vi "Move Stage.vi"(8 "error in (no error)":errorcluster, 9 "Y Axis":dbl, 10 "X Axis":dbl, 11 "2-Axis Stage in":refnum<class "XY Stage Process.lvclass">) -> (0 "error out":errorcluster, 3 "2-Axis Stage out":refnum<class "XY Stage Process.lvclass">)   [LabVIEW 2022 SP3, in "XY Stage Process.lvlib" / "XY Stage Process.lvclass"]
uses:
  XY Stage Process.lvclass
  XY Stage Process.lvclass/XY Stage Process.ctl
  Axis Objects/iMotion Controller/iMotion Controller.lvclass
  Process Framework/Process State Data/Process State Data.lvclass
  <vilib>/ErrorRing/Error Ring.xnode
  <vilib>/Utility/error.llb/Error Cluster From Error Code.vi
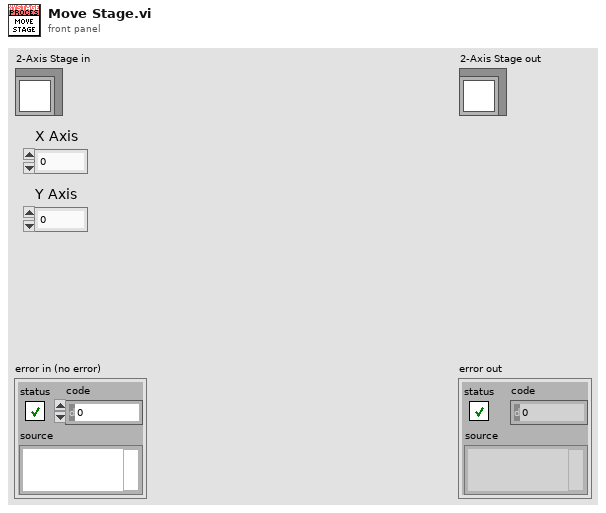
[diagram p1: front panel]
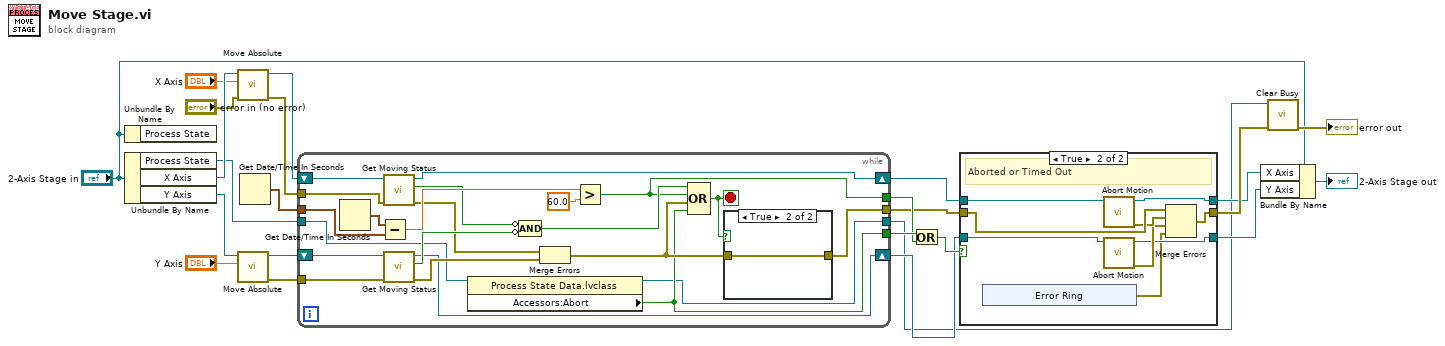
[diagram p0: block diagram]
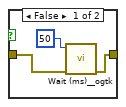
[diagram p3: hidden frame]
diagram:
  n1 = Unbundle By Name("2-Axis Stage in") -> ()  [unwired: 1 out]
  n2 = Unbundle By Name("2-Axis Stage in") -> ("Process State"=w13:refnum<data-value>, "X Axis"=w24:refnum<class "iMotion Controller.lvclass">, "Y Axis"=w23:refnum<class "iMotion Controller.lvclass">)
  n3 = call-dynamic "Move Absolute.vi"("error in (no error)"="error in (no error)", "Desired Position"="X Axis", "iMotion Controller in"=w24) -> ("error out"=w16:errorcluster, "iMotion Controller out"=w18:refnum<class "iMotion Controller.lvclass">)  [unwired: 7 in]
  n4 = call-dynamic "Move Absolute.vi"("Desired Position"="Y Axis", "iMotion Controller in"=w23) -> ("error out"=w15:errorcluster, "iMotion Controller out"=w17:refnum<class "iMotion Controller.lvclass">)  [unwired: 8 in]
  n5 = Get Date/Time In Seconds() -> (seconds since 1Jan1904=w19:timestamp)
  n6 = while {
    tunnel: w16 -> [w34]
    tunnel: [w41] -> w9
    tunnel: w19 -> [w44]
    tunnel: w15 -> [w33]
    tunnel: w13 -> [w30]
    tunnel: [w29] -> w12
    tunnel: [w28] -> w11
    shift-right: [w26] -> w8
    shift-left: w17 -> [w38]
    shift-right: [w27] -> w7
    shift-left: w18 -> [w39]
    tunnel: [w25] -> w1
    stop <- w40 stop-if-true
    n7 = Get Date/Time In Seconds() -> (seconds since 1Jan1904=w45:timestamp)
    n8 = Subtract(x=w45, y=w44) -> (x-y=w42:dbl)
    n9 = call-dynamic "Get Moving Status.vi"("error in (no error)"=w34, "iMotion Controller in"=w39) -> ("error out"=w35:errorcluster, "Moving"=w36:bool, "iMotion Controller out"=w27:refnum<class "iMotion Controller.lvclass">)  [unwired: 7 in]
    n10 = call-dynamic "Get Moving Status.vi"("error in (no error)"=w33, "iMotion Controller in"=w38) -> ("error out"=w32:errorcluster, "Moving"=w37:bool, "iMotion Controller out"=w26:refnum<class "iMotion Controller.lvclass">)  [unwired: 7 in]
    n11 = property class="Process State Data.lvclass"(reference=w30) -> (reference out=w25:refnum<data-value>, "Accessors:Abort"=w29:bool)  [unwired: 1 in, 1 out]
    n12 = Compound Arithmetic op=AND(invert w36, invert w37) -> (w46:bool)
    n13 = Merge Errors(w35, w32) -> (w31:errorcluster)
    n14 = Greater?(x=w42, y=60.0 ("x")) -> (0:w28:bool)
    n15 = Compound Arithmetic op=OR(w46, w28, w31, w29) -> (w40:bool)
    n16 = case shown="True" w40 {
      tunnel: w31 -> [w49 w50]
      tunnel: [w48 w50] -> w41
      frame False {
        n17 = call <userlib>:"Wait (ms)__ogtk.vi"("error in (no error)"=w49, "milliseconds to wait"=u32 50) -> ("error out"=w48:errorcluster)  [unwired: 8 in, 1 out]
      }
      frame True {
      }
    }
  }
  n18 = Or(x=w12, y=w11) -> (x .or. y?=w10:bool)
  n19 = case shown="True" w10 {
    tunnel: w9 -> [w53 w60]
    tunnel: w8 -> [w51 w61]
    tunnel: w7 -> [w52 w62]
    tunnel: [w53 w57] -> w6
    tunnel: [w52 w56] -> w4
    tunnel: [w51 w55] -> w3
    frame False {
    }
    frame True {
      # "Aborted or Timed Out"
      n20 = xnode "Error Ring"() -> ("error out"=w54:errorcluster)
      n21 = call-dynamic "Abort Motion.vi"("iMotion Controller in"=w62) -> ("error out"=w59:errorcluster, "iMotion Controller out"=w56:refnum<class "iMotion Controller.lvclass">)  [unwired: 9 in]
      n22 = call-dynamic "Abort Motion.vi"("iMotion Controller in"=w61) -> ("error out"=w58:errorcluster, "iMotion Controller out"=w55:refnum<class "iMotion Controller.lvclass">)  [unwired: 9 in]
      n23 = Merge Errors(w60, w59, w58, w54) -> (w57:errorcluster)
    }
  }
  n24 = Bundle By Name(cluster="2-Axis Stage in", "X Axis"=w4, "Y Axis"=w3) -> (→"2-Axis Stage out":refnum<class "XY Stage Process.lvclass">)
  n25 = call "Clear Busy.vi"("error in (no error)"=w6, "Process State"=w1) -> ("error out"=→"error out":errorcluster)  [unwired: 8 in, 1 out]
